vi "IgnoreZ1,2,3,5Array.vi"(11 "Zernike Order":i32) -> (3 "output array":i32[](array[numeric]))   [LabVIEW 2020, in "ThorlabsWFS.lvclass"]
uses:
  ThorlabsWFS.lvclass
panel:
  out "initialized array":i32[](array[numeric])
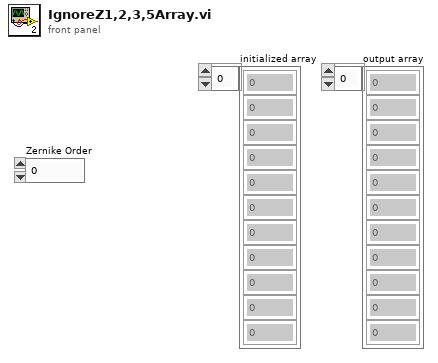
[diagram p1: front panel]
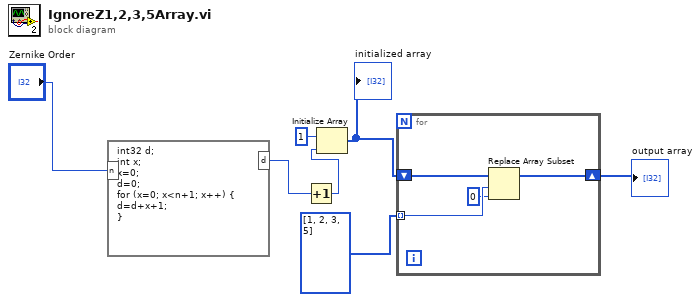
[diagram p0: block diagram]
diagram:
  n1 = formula code="int32 d;\nint x;\nx=0;\nd=0;\nfor (x=0; x<n+1; x++) {\nd=d+x+1;\n}"("n"="Zernike Order") -> ("d"=w5:i32)
  n2 = Increment(x=w5) -> (x+1=w4:i32)
  n3 = Initialize Array(1 ("element"), w4) -> (w1:i32[])
  "initialized array" <- w1
  n4 = for {
    tunnel: i32[] [1, 2, 3, 5] -> [w11] mode=indexing
    shift-right: [w9] -> w2
    shift-left: w1 -> [w8]
    n5 = Replace Array Subset(array=w8, new element=0 ("new element/subarray"), index=w11) -> (w9:i32[])
  }
  "output array" <- w2
